vi "Read Verification CA Bundle Path.vi"(8 "error in (no error)":errorcluster, 11 "SSL Client Context in":refnum<class "SSL Client Context.lvclass">) -> (0 "error out":errorcluster, 2 "Verification CA Bundle Path":path, 3 "SSL Client Context out":refnum<class "SSL Client Context.lvclass">)   [LabVIEW 2013, in "OpenSSL Socket.lvlib" / "SSL Client Context.lvclass"]
uses:
  SSL Client Context.lvclass
  SSL Client Context.lvclass/SSL Client Context.ctl
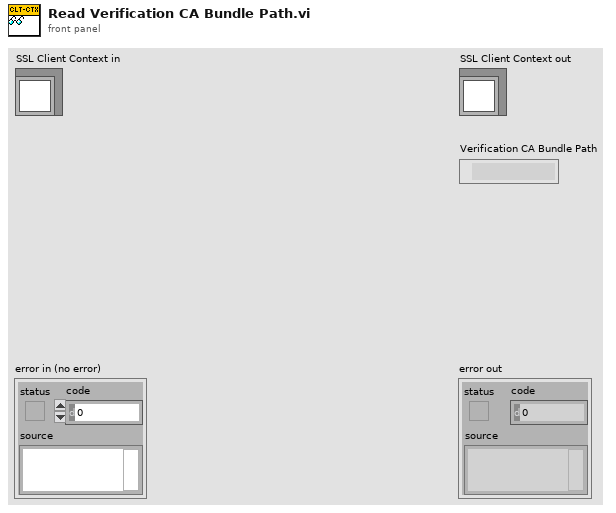
[diagram p1: front panel]
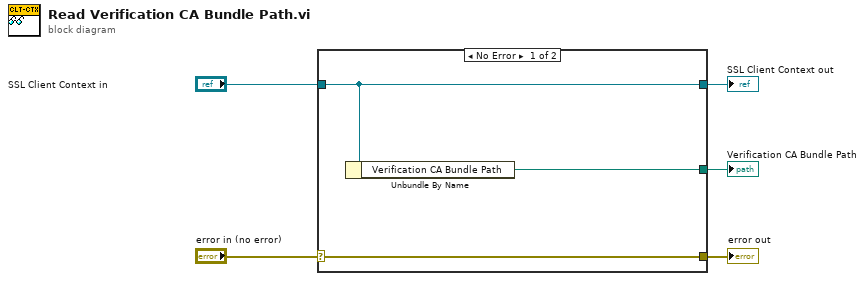
[diagram p0: block diagram]
diagram:
  n1 = case shown="No Error" "error in (no error)" {
    selector: "error in (no error)" -> [w8 w9]
    tunnel: [w8 w9] -> w4
    tunnel: [w7 w10] -> w2
    tunnel: "SSL Client Context in" -> [w7 w10]
    tunnel: [w6 _] -> w1
    frame No Error {
      n2 = Unbundle By Name(w7) -> ("Verification CA Bundle Path"=w6:path)
    }
    frame Error {
    }
  }
  "error out" <- w4
  "SSL Client Context out" <- w2
  "Verification CA Bundle Path" <- w1
